vi "Open.vi"(7 "I2C Channel (0)":u8, 8 "Error In":errorcluster, 9 "Resolution":T8, 10 "I2C Slave Address":T7, 11 "LINX Resource":T1) -> (0 "Error Out":errorcluster, 3 "LINX Resource":T1)   [LabVIEW 2020, in "LMH-LINX.lvlib" / "TCN75A.lvlib"]
doc: "Open the specified I2C channel and initialize the TCN75A."
uses:
  TCN75A.lvlib
  Private/Type Defs/LINX Ref.ctl
  Private/Type Defs/Platform.ctl
  Private/Type Defs/Interface.ctl
  Private/Device/Type Defs/LINX Device Config.ctl
  Private/Device/Type Defs/TCP Config.ctl
  Private/Device/Type Defs/Channels.ctl
  Resolution.ctl
  I2C Address.ctl
  Private/Local IO/LinxI2cWrite.vi
  Utilities/Check Channel.vi
  Private/Utilties/Generate Error.vi
  LMH-LINX.lvlib
  Private/Device/Device.lvlib
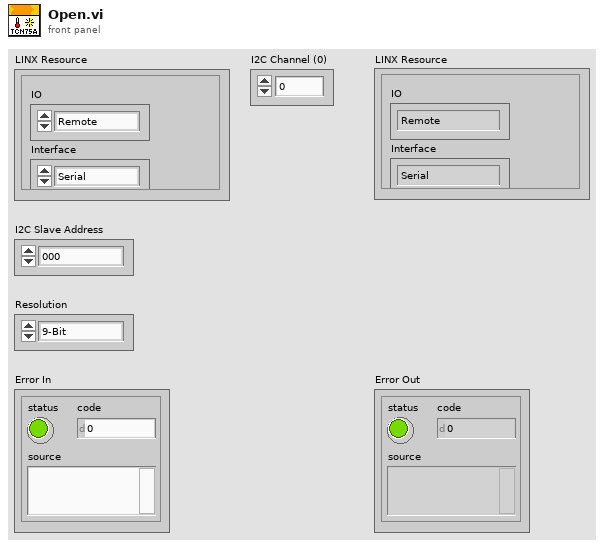
[diagram p1: front panel]
types:
  T1 = typedef "LMH-LINX.lvlib/LINX Ref.ctl" = cluster{"IO":T2, "Interface":T3, "LINX Device Config":T4}
  T2 = typedef "LMH-LINX.lvlib/Platform.ctl" = enum16{"Remote", "Local"}
  T3 = typedef "LMH-LINX.lvlib/Interface.ctl" = enum16{"Serial", "TCP"}
  T4 = typedef "LMH-LINX.lvlib/Device.lvlib/LINX Device Config.ctl" = cluster{"Interface":T3, "COM Port":refnum<visa-resource-name>, "TCP Configuration":T5, "Device Family":u8, "Device ID":u8, "Device Name":string, "TCP Ref":refnum<k5>, "Channels":T6}
  T5 = typedef "LMH-LINX.lvlib/Device.lvlib/TCP Config.ctl" = cluster{"IP Address":string, "Port":u16}
  T6 = typedef "LMH-LINX.lvlib/Channels.ctl" = cluster{"DI":u8[], "DO":u8[], "AI":u8[], "AO":u8[], "PWM":u8[], "QE":u8[], "UART":u8[], "I2C 2":u8[], "SPI":u8[], "CAN":u8[], "Servo":u8[], "AI Ref (V)":dbl, "AI Resolution (Bits)":u8, "AO Ref (V)":dbl, "AO Resolution (Bits)":u8}
  T7 = typedef "LMH-LINX.lvlib/TCN75A.lvlib/I2C Address.ctl" = enum8{"000", "001", "010", "011", "100", "101", "110", "111"}
  T8 = typedef "LMH-LINX.lvlib/TCN75A.lvlib/Resolution.ctl" = enum8{"9-Bit", "10-Bit", "11-Bit", "12-Bit"}
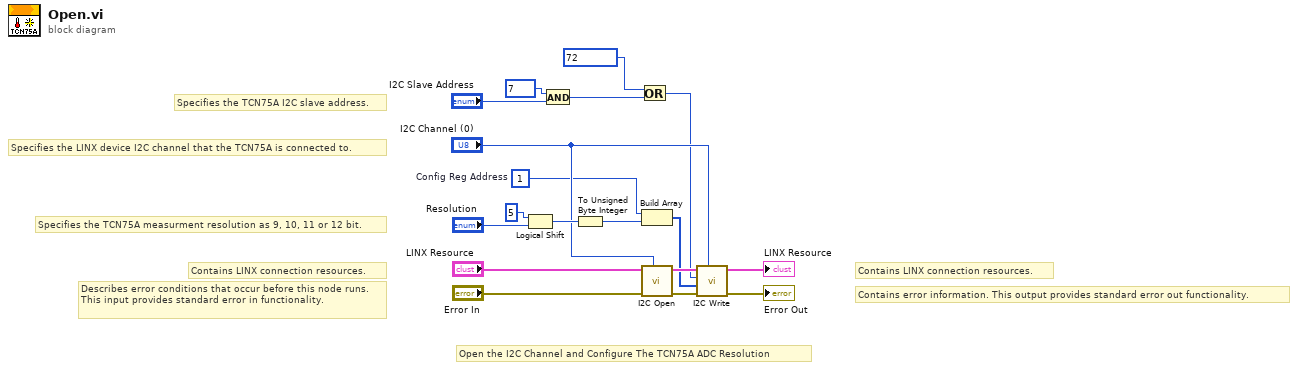
[diagram p0: block diagram]
diagram:
  w5 = u8 1  # Config Reg Address
  # "Specifies the TCN75A measurment resolution as 9, 10, 11 or 12 bit."
  # "Specifies the TCN75A I2C slave address."
  # "Specifies the LINX device I2C channel that the TCN75A is connected to."
  # "Contains LINX connection resources."
  # "Contains error information. This output provides standard error out functionality."
  # "Contains LINX connection resources."
  # "Describes error conditions that occur before this node runs. This input provides standard error in functionality."
  # "Open the I2C Channel and Configure The TCN75A ADC Resolution"
  n1 = Logical Shift(y=i8 5, x="Resolution") -> (x << y=w14:u32)
  n2 = And(x=u8 7, y="I2C Slave Address") -> (x .and. y?=w10:u8)
  n3 = To Unsigned Byte Integer(number=w14) -> (unsigned 8bit integer=w3:u8)
  n4 = Or(x=u8 72, y=w10) -> (x .or. y?=w6:u8)
  n5 = Build Array(w5, w3) -> (w4:u8[])
  n6 = call "I2C Open.vi"("I2C Channel (0)"="I2C Channel (0)", "Error In"="Error In", "LINX Resource"="LINX Resource") -> ("Error Out"=w8:errorcluster, "LINX Resource"=w9:T1)  [unwired: 7 in]
  n7 = call "I2C Write.vi"("I2C Channel"="I2C Channel (0)", "Error In"=w8, "Data"=w4, "I2C Slave Address (0)"=w6, "LINX Resource"=w9) -> ("Error Out"=→"Error Out":errorcluster, "LINX Resource"=→"LINX Resource":T1)  [unwired: 5 in]
